vi "Decode.vi"(10 "Encoded String":string, 11 "CfgEncoding in":refnum<class "Encoding.Base64.lvclass">) -> (2 "String":string, 3 "CfgEncoding out":refnum<class "Encoding.Base64.lvclass">)   [LabVIEW 2013, in "SMOConfig.lvlib" / "Encoding.Base64.lvclass"]
uses:
  Encoding.Base64.lvclass
  <vilib>/httpClient/LabVIEWHTTPClient.lvlib
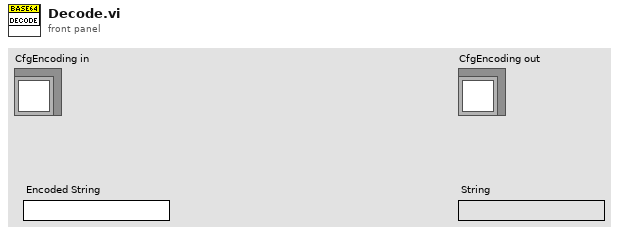
[diagram p1: front panel]
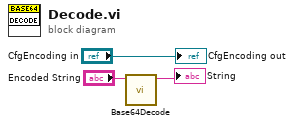
[diagram p0: block diagram]
diagram:
  n1 = call <vilib>:"Base64Decode.vi"("buffer in"="Encoded String") -> ("decoded string"=→"String":string)  [unwired: 9 in, 1 out]
  "CfgEncoding out" <- "CfgEncoding in"
